vi "Ready to run.vi"(8 "error in (no error)":errorcluster, 11 "ZenGage v3.0 UI in":T1) -> (0 "error out":errorcluster, 3 "ZenGage v3.0 UI out":T1)   [LabVIEW 2019, in "ZenGage v3.0 UI.lvclass"]
uses:
  ZenGage v3.0 UI.lvclass
  Type Definitions/General/UI States(UI button enable disable).ctl
  Type Definitions/JSON Read/UI JSON read cluster.ctl
  Type Definitions/General/JSONRead.ctl
  Type Definitions/Inspection/Inspection Cluster.ctl
  Type Definitions/Diagnostics/Diagnostics(Cluster).ctl
  Type Definitions/Edit tolerance settings/Rack Selection.ctl
  <vilib>/Utility/miscctls.llb/LVPoint32TypeDef.ctl
  Type Definitions/Edit tolerance settings/Edit Tolerance Input.ctl
  Type Definitions/Edit tolerance settings/Edit Tolerance Overall Cluster.ctl
  Type Definitions/Controls and Indicators/Select a part (combobox).ctl
  Type Definitions/Controls and Indicators/EDL control references.ctl
  Type Definitions/Controls and Indicators/Diagnostics control referencs.ctl
  Type Definitions/Controls and Indicators/Inspection control references.ctl
  Type Definitions/Controls and Indicators/General_Control references.ctl
  Type Definitions/Controls and Indicators/Controls and Indicators Cluster.ctl
  Common/Controls/Pop-up Input.ctl
  Type Definitions/General/UIDataCluster.ctl
  Type Definitions/General/Master sample references.ctl
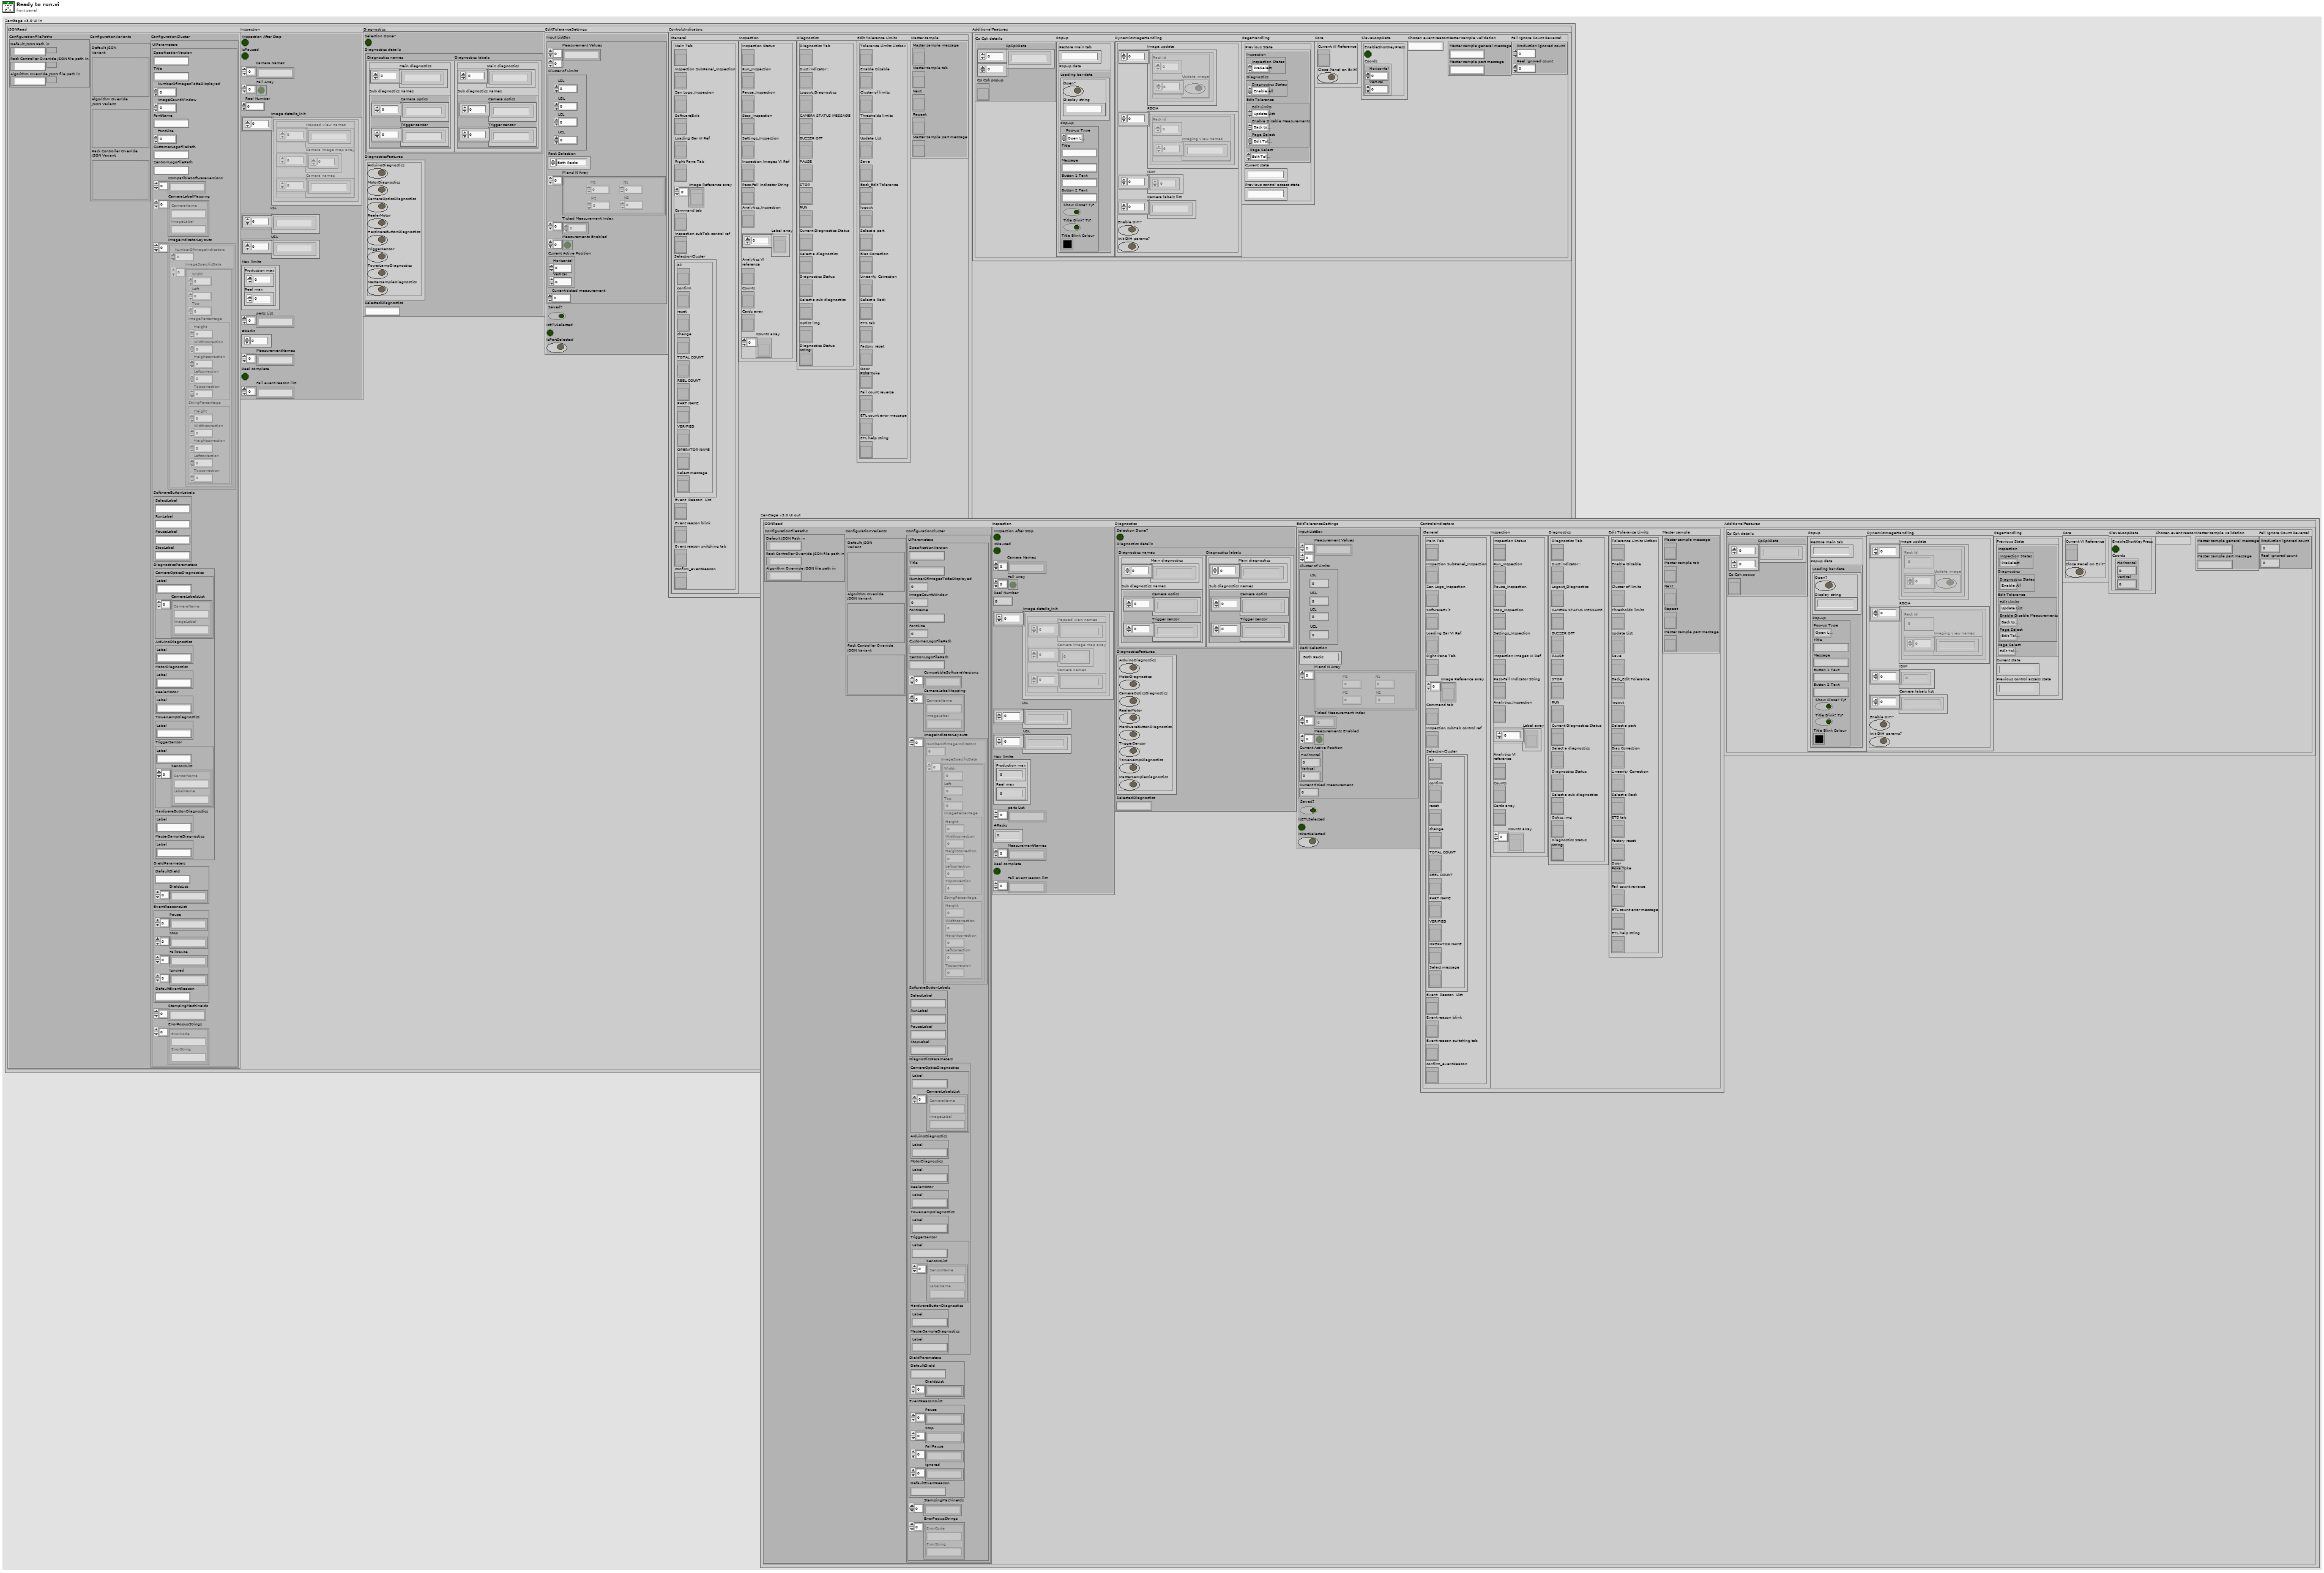
[diagram p1: front panel]
types:
  T1 = typedef "UIDataCluster.ctl" = cluster{"JSONRead":T2, "Inspection":T4, "Diagnostics":T5, "EditToleranceSettings":T6, "ControlsIndicators":T10, "AdditionalFeatures":cluster{"Cp Cpk details":cluster{"CpCpkData":string[][], "Cp Cpk popup":refnum<vi>}, "Popup":cluster{"Restore main tab":string, "Popup data":cluster{"Loading bar data":cluster{"Open?":bool, "Display string":string}, "Pop-up":T16}}, "DynamicImageHandling":cluster{"Image update":cluster{"Rack Id":i32, "Update image":bool[]}[], "RBCIA":cluster{"Rack Id":u8, "Imaging view names":string[]}[], "ISIM":u8[], "Camera labels list":string[], "Enable DIH?":bool, "Init DIH params?":bool}, "PageHandling":cluster{"Previous State":T17, "Current state":string, "Previous control access state":string}, "Core":cluster{"Current VI Reference":refnum<vi>, "Close Panel on Exit?":bool}, "SlaveLoopData":cluster{"EnableShortKeyPress":bool, "Point32":T9}, "Chosen event reason":string, "Master sample validation":cluster{"Master sample general message":string, "Master sample part message":string}, "Fail Ignore Count Reversal":cluster{"Production ignored count":u64, "Reel ignored count":u64}}}
  T2 = typedef "ZenGage v3.0 UI.lvclass/JSONRead.ctl" = cluster{"ConfigurationFilePaths":cluster{"Default JSON Path in":path, "Rack Controller Override JSON file path in":path, "Algorithm Overrride JSON file path in ":path}, "ConfigurationVariants":cluster{"Default JSON \nVariant":variant, "Algorithm Override\nJSON Variant":variant, "Rack Controller Override\nJSON Variant":variant}, "ConfigurationCluster":T3}
  T3 = typedef "ZenGage v3.0 UI.lvclass/UI JSON read cluster.ctl" = cluster{"UIParameters":cluster{"SpecificationVersion":string, "Title":string, "NumberOfImagesToBeDisplayed":dbl, "ImageCountWindow":dbl, "FontName":string, "FontSize":dbl, "CustomerLogoFilePath":string, "ZentronLogoFilePath":string, "CompatibleSoftwareVersions":string[], "CameraLabelMapping":cluster{"CameraName":string, "ImageLabel":string}[], "ImageIndicatorLayouts":cluster{"NumberOfImageIndicators":dbl, "ImageSpecificData":cluster{"Width":dbl, "Left":dbl, "Top":dbl, "ImagePercentage":cluster{"Height":dbl, "Widthcorrection":i64, "Heightcorrection":i64, "Leftcorrection":dbl, "Topcorrection":dbl}, "StringPercentage":cluster{"Height":dbl, "Widthcorrection":i64, "Heightcorrection":dbl, "Leftcorrection":dbl, "Topcorrection":dbl}}[]}[], "SoftwareButtonLabels":cluster{"SelectLabel":string, "RunLabel":string, "PauseLabel":string, "StopLabel":string}, "DiagnosticsParameters":cluster{"CameraOpticsDiagnostics":cluster{"Label":string, "CameraLabelsList":cluster{"CameraName":string, "ImageLabel":string}[]}, "ArduinoDiagnostics":cluster{"Label":string}, "MotorDiagnostics":cluster{"Label":string}, "ReelerMotor":cluster{"Label":string}, "TowerLampDiagnostics":cluster{"Label":string}, "TriggerSensor":cluster{"Label":string, "SensorsList":cluster{"SensorName":string, "LabelName":string}[]}, "HardwareButtonDiagnostics":cluster{"Label":string}, "MasterSampleDiagnostics":cluster{"Label":string}}, "DieIdParameters":cluster{"DefaultDieId":string, "DieIdsList":string[]}, "EventReasonsList":cluster{"Pause":string[], "Stop":string[], "FailPause":string[], "Ignored":string[], "DefaultEventReason":string}, "StampingMachineIds":string[], "ErrorPopupStrings":cluster{"ErrorCode":string, "ErrorString":string}[]}}
  T4 = typedef "ZenGage v3.0 UI.lvclass/Inspection Cluster.ctl" = cluster{"Inspection After Stop":bool, "IsPaused":bool, "Camera Names":string[], "Fail Array":bool[], "Reel Number":u32, "Image details_init":cluster{"Mapped view names":string[], "Camera image map array":i32[], "Camera names":string[]}[], "LSL":string[], "USL":string[], "Max limits":cluster{"Production max":u64, "Reel max":u64}, "parts List":string[], "#Racks":u8, "MeasurementNames":string[], "Reel complete":bool, "Fail event reason list":string[]}
  T5 = typedef "ZenGage v3.0 UI.lvclass/Diagnostics(Cluster).ctl" = cluster{"Selection Done?":bool, "Diagnostics details":cluster{"Diagnostics names":cluster{"Main diagnostics":string[], "Sub diagnostics names":cluster{"Camera optics":string[], "Trigger sensor":string[]}}, "Diagnostics labels":cluster{"Main diagnostics":string[], "Sub diagnostics names":cluster{"Camera optics":string[], "Trigger sensor":string[]}}}, "DiagnosticsFeatures":cluster{"ArduinoDiagnostics":bool, "MotorDiagnostics":bool, "CameraOpticsDiagnostics":bool, "ReelerMotor":bool, "HardwareButtonDiagnostics":bool, "TriggerSensor":bool, "TowerLampDiagnostics":bool, "MasterSampleDiagnostics":bool}, "SelectedDiagnostics":string}
  T6 = typedef "ZenGage v3.0 UI.lvclass/Edit Tolerance Overall Cluster.ctl" = cluster{"Input ListBox":T7, "Saved?":bool, "IsETLSelected":bool, "IsPartSelected":bool}
  T7 = typedef "ZenGage v3.0 UI.lvclass/Edit Tolerance Input.ctl" = cluster{"Measurement Values":string[][], "Cluster of Limits":cluster{"LSL":dbl, "USL":dbl, "LCL":dbl, "UCL":dbl}, "Rack Selection":T8, "M and N Array":cluster{"M1":u64, "M2":u64, "N1":u64, "N2":u64}[], "Ticked Measurement Index":u32[], "Measurements Enabled":bool[], "Current Active Position":T9, "Current ticked measurement":dbl}
  T8 = typedef "ZenGage v3.0 UI.lvclass/Rack Selection.ctl" = enum16{"Both Racks", "Rack 2", "Rack 1"}
  T9 = typedef "LVPoint32TypeDef.ctl" = cluster{"Horizontal":i32, "Vertical":i32}
  T10 = typedef "ZenGage v3.0 UI.lvclass/Controls and Indicators Cluster.ctl" = cluster{"General":T11, "Inspection":T12, "Diagnostics":T13, "Edit Tolerance Limits":T14, "Master sample":T15}
  T11 = typedef "ZenGage v3.0 UI.lvclass/General_Control references.ctl" = cluster{"Main Tab":refnum<vi>, "Inspection SubPanel_Inspection":refnum<vi>, "Zen Logo_Inspection":refnum<vi>, "SoftwareExit":refnum<vi>, "Loading Bar VI Ref":refnum<vi>, "Right Pane Tab":refnum<vi>, "Image Reference array":refnum<vi>[], "Command tab":refnum<vi>, "Inspection subTab control ref":refnum<vi>, "SelectionCluster":cluster{"ok":refnum<vi>, "confirm":refnum<vi>, "reset":refnum<vi>, "change":refnum<vi>, "TOTAL COUNT":refnum<vi>, "REEL COUNT":refnum<vi>, "PART NAME":refnum<vi>, "VERIFIED":refnum<vi>, "OPERATOR NAME":refnum<vi>, "Select message":refnum<vi>}, "Event  Reason  List":refnum<vi>, "Event reason blink":refnum<vi>, "Event reason switching tab":refnum<vi>, "confirm_eventReason":refnum<vi>}
  T12 = typedef "ZenGage v3.0 UI.lvclass/Inspection control references.ctl" = cluster{"Inspection Status":refnum<vi>, "Run_Inspection":refnum<vi>, "Pause_Inspection":refnum<vi>, "Stop_Inspection":refnum<vi>, "Settings_Inspection":refnum<vi>, "Inspection Images VI Ref":refnum<vi>, "Pass-Fail Indicator String":refnum<vi>, "Analytics_Inspection":refnum<vi>, "Label array":refnum<vi>[], "Analytics VI\nreference":refnum<vi>, "Counts":refnum<vi>, "Cards array":refnum<vi>, "Counts array":refnum<vi>[]}
  T13 = typedef "ZenGage v3.0 UI.lvclass/Diagnostics control referencs.ctl" = cluster{"Diagnostics Tab":refnum<vi>, "Dust indicator :":refnum<vi>, "Logout_Diagnostics":refnum<vi>, "CAMERA STATUS MESSAGE":refnum<vi>, "BUZZER OFF":refnum<vi>, "PAUSE":refnum<vi>, "STOP":refnum<vi>, "RUN":refnum<vi>, "Current Diagnostics Status":refnum<vi>, "Select a diagnostics":refnum<vi>, "Diagnostics Status":refnum<vi>, "Select a sub diagnostics":refnum<vi>, "Optics img":refnum<vi>, "Diagnostics Status\nString":refnum<vi>}
  T14 = typedef "ZenGage v3.0 UI.lvclass/EDL control references.ctl" = cluster{"Tolerance Limits Listbox":refnum<vi>, "Enable Disable":refnum<vi>, "Cluster of limits":refnum<vi>, "Thresholds limits":refnum<vi>, "Update List":refnum<vi>, "Save":refnum<vi>, "Back_Edit Tolerance":refnum<vi>, "logout":refnum<vi>, "Select a part":refnum<vi>, "Bias Correction":refnum<vi>, "Linearity Correction":refnum<vi>, "Select a Rack":refnum<vi>, "ETS tab":refnum<vi>, "Factory reset":refnum<vi>, "Door\nPoka Yoke":refnum<vi>, "Fail count reverse":refnum<vi>, "ETL count error message":refnum<vi>, "ETL help string":refnum<vi>}
  T15 = typedef "Master sample references.ctl" = cluster{"Master sample message":refnum<vi>, "Master sample tab":refnum<vi>, "Next":refnum<vi>, "Repeat":refnum<vi>, "Master sample part message":refnum<vi>}
  T16 = typedef "Pop-up Input.ctl" = cluster{"Pop-up Type":enum16{"Open Logo Display", "Close Logo Display", "Open Loading Bar", "Close Loading Bar", "Open Alert Display", "Close Alert Display", "One button dialog box", "Two button dialog box", "User Authentication"}, "Title":string, "Message":string, "Button 1 Text":string, "Button 2 Text":string, "Show Close? T/F":bool, "Title Blink? T/F":bool, "Title Blink Colour":u32}
  T17 = typedef "ZenGage v3.0 UI.lvclass/UI States(UI button enable disable).ctl" = cluster{"Inspection":cluster{"Inspection States":enum16{"PreSelect", "Back _Inspection", "Analytics", "Ready To Run", "Ready To Insert", "Enable All buttons", "Disable All Buttons", "Settings", "Select", "Stop", "Pause", "Inspect"}}, "Diagnostics":cluster{"Diagnostics States":enum16{"Enable All", "Camera Optics Fail", "Loading Bar", "Camera Optics", "Motor", "Arduino", "POST Done", "POST"}}, "Edit Tolerance":cluster{"Edit Limits":enum16{"Update List"}, "Enable Disable Measurements":enum16{"Back to Edit Tolerance"}, "Page Select":enum16{"Edit Tolerance Limits", "Enable Disable Buttons"}}, "Page Select":enum16{"Edit Tolerance", "Diagnostics", "Inspection"}}
  T18 = enum8{"Enabled", "Disabled", "Disabled and Grayed Out"}
  T19 = enum32{"Analytics", "Blank", "Diagnostics", "Run", "Edit Tolerance Settings"}
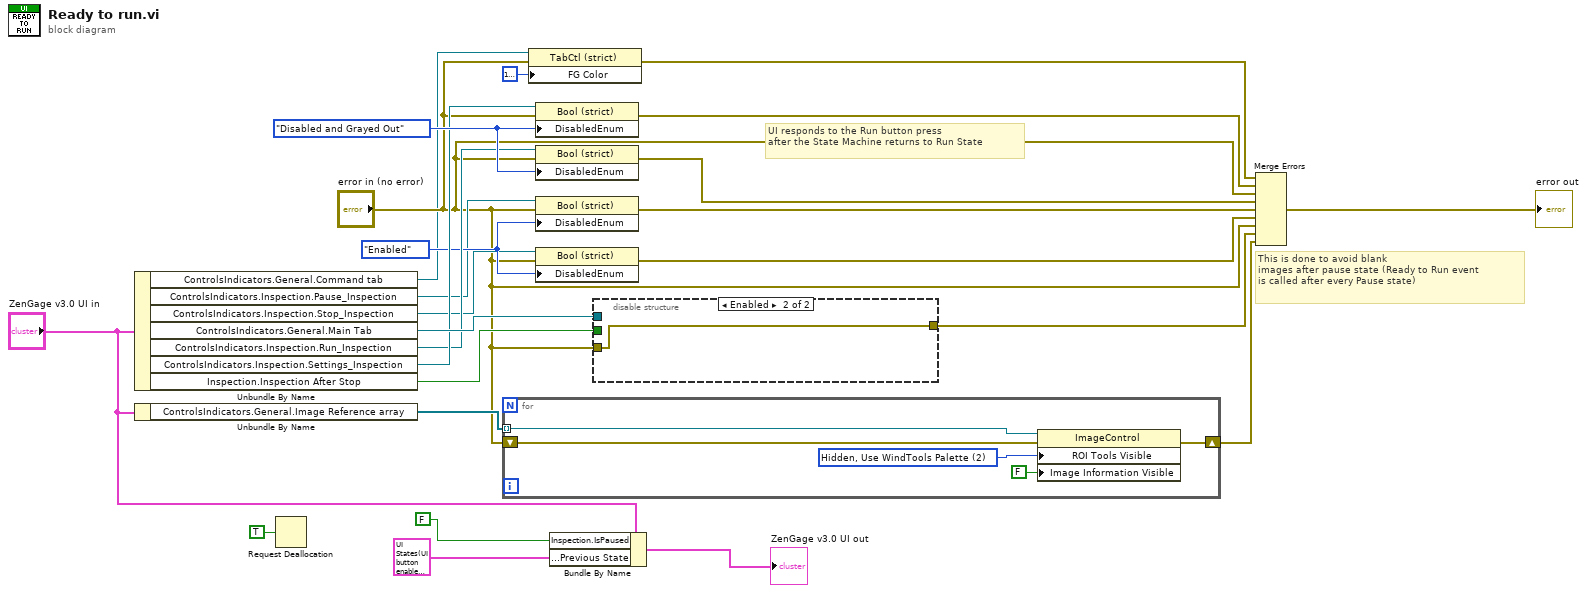
[diagram p0: block diagram]
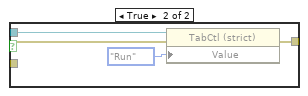
[diagram p3: hidden frame]
diagram:
  w24 = T18."Disabled and Grayed Out" ("Disabled")
  w12 = T18."Enabled" ("Disabled")
  # "This is done to avoid blank\nimages after pause state (Ready to Run event\nis called after every Pause state)"
  # "UI responds to the Run button press\nafter the State Machine returns to Run State"
  n1 = Unbundle By Name("ZenGage v3.0 UI in") -> ("ControlsIndicators.General.Command tab"=w3:refnum<vi>, "ControlsIndicators.Inspection.Pause_Inspection"=w11:refnum<vi>, "ControlsIndicators.Inspection.Stop_Inspection"=w10:refnum<vi>, "ControlsIndicators.General.Main Tab"=w22:refnum<vi>, "ControlsIndicators.Inspection.Run_Inspection"=w17:refnum<vi>, "ControlsIndicators.Inspection.Settings_Inspection"=w21:refnum<vi>, "Inspection.Inspection After Stop"=w23:bool)
  n2 = Unbundle By Name("ZenGage v3.0 UI in") -> ("ControlsIndicators.General.Image Reference array"=w19:refnum<vi>[])
  n3 = Request Deallocation(TRUE ("flag")) -> ()
  n4 = for {
    tunnel: w19 -> [w30] mode=indexing
    shift-right: [w27] -> w20
    shift-left: "error in (no error)" -> [w28]
    w29 = u32 2 items=["Visible", "Hidden", "Hidden, Use WindTools Palette"] ("ROI Tools Visible")
    n5 = property class="ImageControl"(reference=w30, error in=w28, "ROI Tools Visible"=w29, "Image Information Visible"=FALSE) -> (error out=w27:errorcluster)  [unwired: 1 out]
  }
  n6 = property class="TabCtl (strict)"(reference=w3, error in="error in (no error)", "FG Color"=u32 16777216) -> (error out=w1:errorcluster)  [unwired: 1 out]
  n7 = property class="Bool (strict)"(reference=w21, error in="error in (no error)", "DisabledEnum"=w24) -> (error out=w25:errorcluster)  [unwired: 1 out]
  n8 = property class="Bool (strict)"(reference=w17, error in="error in (no error)", "DisabledEnum"=w24) -> (error out=w18:errorcluster)  [unwired: 1 out]
  n9 = property class="Bool (strict)"(reference=w11, error in="error in (no error)", "DisabledEnum"=w12) -> (error out=w13:errorcluster)  [unwired: 1 out]
  n10 = property class="Bool (strict)"(reference=w10, error in="error in (no error)", "DisabledEnum"=w12) -> (error out=w14:errorcluster)  [unwired: 1 out]
  n11 = Bundle By Name(cluster="ZenGage v3.0 UI in", "Inspection.IsPaused"=FALSE ("Inspection.Paused?"), "AdditionalFeatures.PageHandling.Previous State"=T17 {"Inspection"={"Inspection States"=enum."Ready To Run"}, "Diagnostics"={"Diagnostics States"=enum."Enable All"}, "Edit Tolerance"={"Edit Limits"=enum."Update List", "Enable Disable Measurements"=enum."Back to Edit Tolerance", "Page Select"=enum."Edit Tolerance Limits"}, "Page Select"=enum."Inspection"} ("UI States")) -> (→"ZenGage v3.0 UI out":T1)
  n12 = disable-structure shown="Enabled" {
    disable-tunnel: w23 -> [w34 _]
    disable-tunnel: w22 -> [w33 _]
    disable-tunnel: [w32 w40] -> w16
    disable-tunnel: "error in (no error)" -> [w31 w40]
    frame Disabled {
      n13 = case shown="False" w34 {
        tunnel: [w35 w39] -> w32
        tunnel: w33 -> [_ w37]
        tunnel: w31 -> [w35 w36]
        frame False {
        }
        frame True {
          n14 = property class="TabCtl (strict)"(reference=w37, error in=w36, "Value"=T19."Run") -> (error out=w39:errorcluster)  [unwired: 1 out]
        }
      }
    }
    frame Enabled {
    }
  }
  n15 = Merge Errors(w1, w25, "error in (no error)", w18, w13, w14, "error in (no error)", w16, w20) -> (→"error out":errorcluster)
